vi "Set_CtlValueSGNL.vi"(8 "error in (no error)":errorcluster, 9 "Value":variant, 10 "Control Label":string, 11 "CtlLookup In":T1) -> (0 "error out":errorcluster, 3 "CtlLookup Out":T1)   [LabVIEW 2020, in "CtlReferences.lvlib" / "CtlReferences.lvclass"]
doc: "This VI uses the GetControlByReference to Set the Value (signalling) of the specified control as a variant"
uses:
  CtlReferences.lvclass
  TypeDefs/CtlLookup.ctl
  CtlReferences.lvclass/CtlReferences.ctl
  GetControlRef/GetControl_Control.vi
  GetControlRef/GetCtlRef_Wrap.vi
  GetCtlRef.vi
  <vilib>/Utility/error.llb/Error Cluster From Error Code.vi
  Error_ToSpecificClass.vi
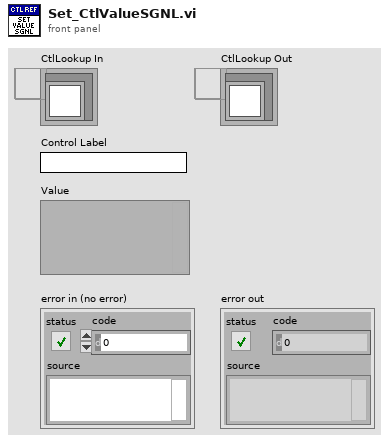
[diagram p1: front panel]
types:
  T1 = typedef "CtlReferences.lvlib/CtlReferences.lvclass/CtlLookup.ctl" = refnum<data-value>
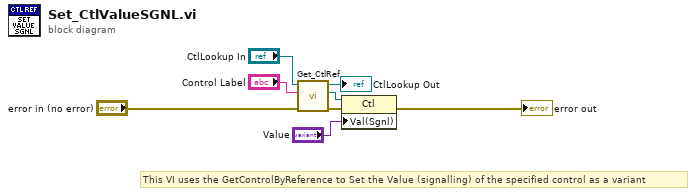
[diagram p0: block diagram]
diagram:
  # "This VI uses the GetControlByReference to Set the Value (signalling) of the specified control as a variant"
  n1 = call-poly "Get_CtlRef.vi"("error in (no error)"="error in (no error)", "Control Label"="Control Label", "CtlLookup In"="CtlLookup In") -> ("error out"=w5:errorcluster, "Reference Out"=w4:refnum<vi>, "CtlLookup Out"=→"CtlLookup Out":T1)  [unwired: 6 in]
  n2 = property class="Ctl"(reference=w4, error in=w5, "Val(Sgnl)"="Value") -> (error out=→"error out":errorcluster)  [unwired: 1 out]
